vi "PolyFit0to-60_1.vi"(11 "input variable":dbl) -> (3 "output variable":dbl)   [LabVIEW 2022 SP3]
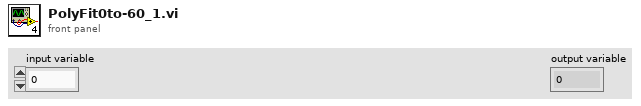
[diagram p1: front panel]
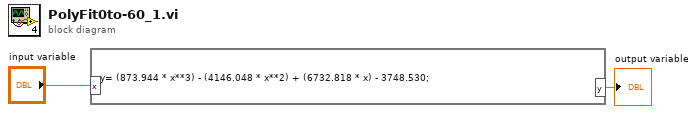
[diagram p0: block diagram]
diagram:
  n1 = formula code="y= (873.944 * x**3) - (4146.048 * x**2) + (6732.818 * x) - 3748.530;"("x"="input variable") -> ("y"=→"output variable":dbl)
